vi "SimpleGit-Push.vi"(11 "path":path) -> ()   [LabVIEW 2017]
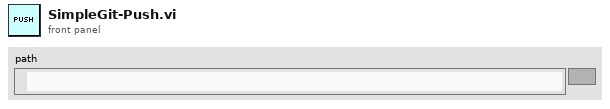
[diagram p1: front panel]
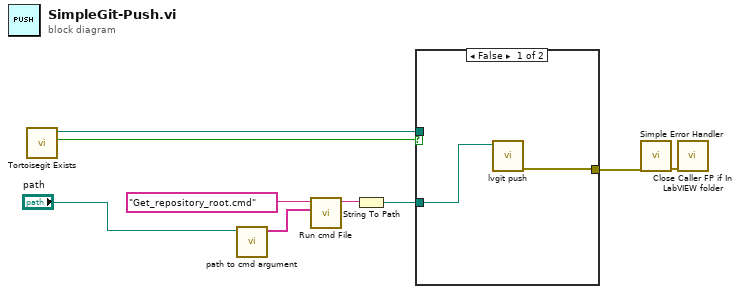
[diagram p0: block diagram]
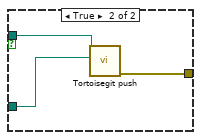
[diagram p2: hidden frame]
diagram:
  n1 = call "Tortoisegit Exists.vi"() -> ("file or folder exists?"=w8:bool, "TortoiseGitProc.exe"=w7:path)  [unwired: 10 in]
  n2 = call "path to cmd argument.vi"("path"="path") -> ("Array"=w5:string[])  [unwired: 10 in]
  n3 = call "Run cmd File.vi"("args"=w5, "name or relative path"="Get_repository_root.cmd") -> ("standard output"=w3:string)  [unwired: 7 in, 2 out]
  n4 = String To Path(string=w3) -> (path=w1:path)
  n5 = case shown="False" w8 {
    tunnel: w7 -> [_ w13]
    tunnel: w1 -> [w11 w14]
    tunnel: [w10 w12] -> w6
    frame False {
      n6 = call "lvgit push.vi"("path"=w11) -> ("error out"=w10:errorcluster)  [unwired: 10 in]
    }
    frame True {
      n7 = call "Tortoisegit push.vi"("path"=w14, "TortoiseGitProc.exe"=w13) -> ("error out"=w12:errorcluster)  [unwired: 9 in]
    }
  }
  n8 = call <vilib>:"Simple Error Handler.vi"("error in (no error)"=w6) -> ("error out"=w9:errorcluster)  [unwired: 4 in, 4 out]
  n9 = call "Close Caller FP if In LabVIEW folder.vi"("error in (no error)"=w9) -> ()  [unwired: 10 in, 1 out]
